vi "Host - sender.vi"() -> ()   [LabVIEW 2017]
panel:
  out "decimal integer string":string
  in  "stop":bool
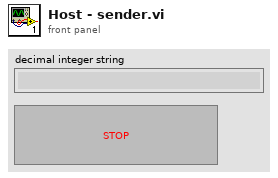
[diagram p1: front panel]
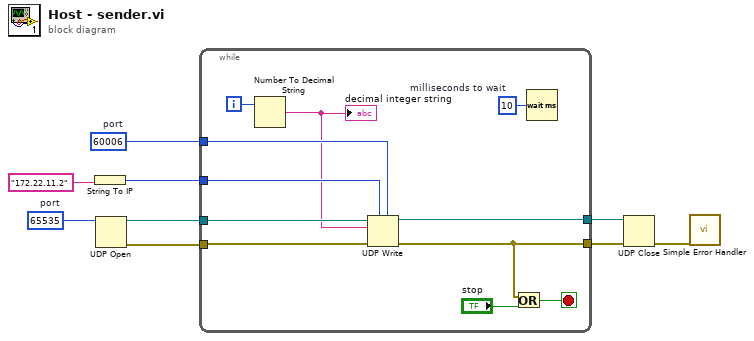
[diagram p0: block diagram]
diagram:
  w4 = u16 60006  # port
  w9 = u16 65535  # port
  n1 = String To IP(1:"172.22.11.2") -> (0:w5:u32)
  n2 = UDP Open(11:w9) -> (port=w7:refnum<k16>, 0:w8:errorcluster)  [unwired: 4 in, 1 out]
  n3 = while {
    tunnel: w8 -> [w18]
    tunnel: w7 -> [w19]
    tunnel: w5 -> [w17]
    tunnel: w4 -> [w16]
    tunnel: [w13] -> w3
    tunnel: [w11] -> w2
    i -> [w15]
    stop <- w12 stop-if-true
    w20 = u32 10  # milliseconds to wait
    n4 = Number To Decimal String(number=w15) -> (decimal integer string=w14:string)  [unwired: 1 in]
    "decimal integer string" <- w14
    n5 = UDP Write(address=w17, port or service name=w16, connection ID=w19, data in=w14, 8:w18) -> (error out=w11:errorcluster, 3:w13:refnum<k16>)  [unwired: 1 in]
    n6 = Or(x=w11, y="stop") -> (x .or. y?=w12:bool)
    n7 = Wait (ms)(milliseconds to wait=w20) -> ()  [unwired: 1 out]
  }
  n8 = UDP Close(connection ID=w3, 8:w2) -> (error out=w1:errorcluster)  [unwired: 1 out]
  n9 = call <vilib>:"Simple Error Handler.vi"("error in (no error)"=w1) -> ()  [unwired: 4 in, 5 out]
